vi "set_watchdog.vi"(7 "set watchdog on/off (F)":bool, 8 "error in (no error)":errorcluster, 10 "set timer":dbl[unit], 11 "LightSourceMH110124MaiTai in":refnum<class "LightSourceMH110124MaiTai.lvclass">) -> (0 "error out":errorcluster, 3 "LightSourceMH110124MaiTai out":refnum<class "LightSourceMH110124MaiTai.lvclass">)   [LabVIEW 2010, in "LightSourceMH110124MaiTai.lvclass"]
uses:
  LightSourceMH110124MaiTai.lvclass
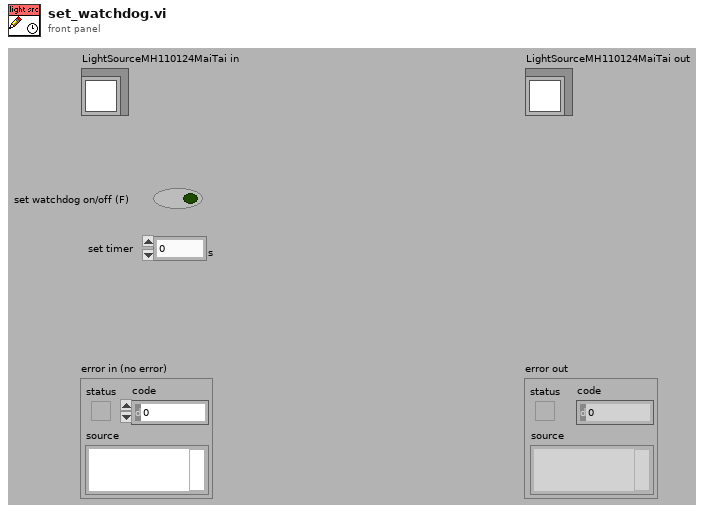
[diagram p1: front panel]
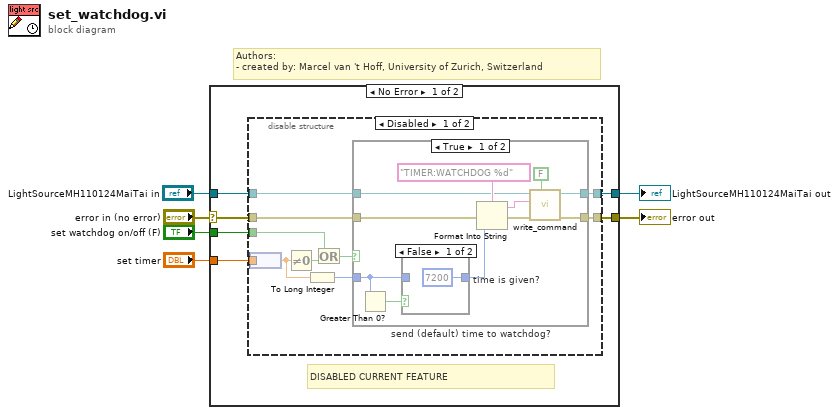
[diagram p0: block diagram]
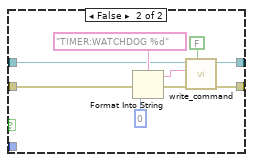
[diagram p3: hidden frame]
diagram:
  # "Authors: \n- created by: Marcel van 't Hoff, University of Zurich, Switzerland"
  n1 = case shown="No Error" "error in (no error)" {
    selector: "error in (no error)" -> [w11 w48]
    tunnel: [w10 w48] -> w5
    tunnel: [w7 w47] -> w4
    tunnel: "LightSourceMH110124MaiTai in" -> [w12 w47]
    tunnel: "set watchdog on/off (F)" -> [w9 _]
    tunnel: "set timer" -> [w8 _]
    frame No Error {
      # "DISABLED CURRENT FEATURE"
      n2 = disable-structure shown="Disabled" {
        disable-tunnel: w12 -> [w22 w46]
        disable-tunnel: w11 -> [w21 w45]
        disable-tunnel: [w20 w45] -> w10
        disable-tunnel: w9 -> [w19 _]
        disable-tunnel: w8 -> [w16 _]
        disable-tunnel: [w13 w46] -> w7
        frame Disabled {
          n3 = node(w16) -> (w15:dbl)
          n4 = Not Equal To 0?(x=w15) -> (x != 0?=w18:bool)
          n5 = To Long Integer(number=w15) -> (32bit integer=w14:i32)
          n6 = Or(x=w19, y=w18) -> (x .or. y?=w17:bool)
          n7 = case "send (default) time to watchdog?" shown="True" w17 {
            tunnel: w22 -> [w26 w40]
            tunnel: w21 -> [w31 w44]
            tunnel: [w27 w41] -> w20
            tunnel: w14 -> [w32 _]
            tunnel: [w25 w39] -> w13
            frame True {
              n8 = Greater Than 0?(x=w32) -> (x > 0?=w33:bool)
              n9 = case "time is given?" shown="False" w33 {
                tunnel: w32 -> [_ w35]
                tunnel: [7200 ("set timer") w35] -> w30
                frame False {
                }
                frame True {
                }
              }
              n10 = Format Into String(format string="TIMER:WATCHDOG %d", error in=w31, w30) -> (resulting string=w23:string, error out=w28:errorcluster)  [unwired: 1 in]
              n11 = call-dynamic "write_command.vi"("read (T)"=FALSE, "error in (no error)"=w28, "string to write"=w23, "LightSourceMH110124MaiTai in"=w26) -> ("error out"=w27:errorcluster, "LightSourceMH110124MaiTai out"=w25:refnum<class "LightSourceMH110124MaiTai.lvclass">)  [unwired: 5 in, 1 out]
            }
            frame False {
              n12 = Format Into String(format string="TIMER:WATCHDOG %d", error in=w44, 0 ("input 1")) -> (resulting string=w37:string, error out=w42:errorcluster)  [unwired: 1 in]
              n13 = call-dynamic "write_command.vi"("read (T)"=FALSE, "error in (no error)"=w42, "string to write"=w37, "LightSourceMH110124MaiTai in"=w40) -> ("error out"=w41:errorcluster, "LightSourceMH110124MaiTai out"=w39:refnum<class "LightSourceMH110124MaiTai.lvclass">)  [unwired: 5 in, 1 out]
            }
          }
        }
        frame Enabled {
        }
      }
    }
    frame Error {
    }
  }
  "error out" <- w5
  "LightSourceMH110124MaiTai out" <- w4
